vi "Get Filter Configuration String.vi"(11 "Base Filter in":refnum<class "Base Filter.lvclass">) -> (2 "Filter Configuration":string)   [LabVIEW 2016, in "Assert API Components.lvlib" / "Base Filter.lvclass"]
uses:
  Base Filter.lvclass
  Base Filter.lvclass/Base Filter.ctl
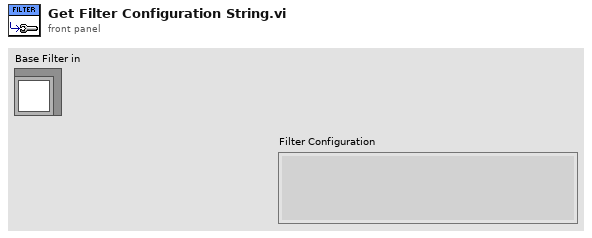
[diagram p1: front panel]
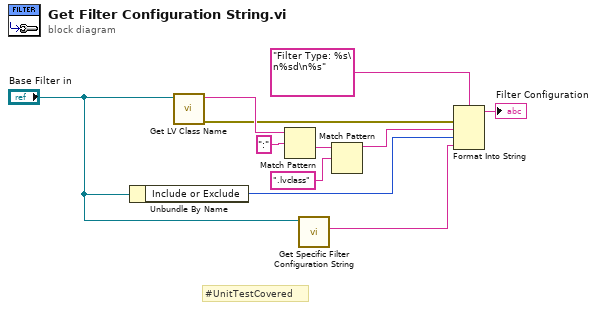
[diagram p0: block diagram]
diagram:
  # "#UnitTestCovered"
  n1 = Unbundle By Name("Base Filter in") -> ("Include or Exclude"=w3:enum16{"Include", "Exclude"})
  n2 = call <vilib>:"Get LV Class Name.vi"("object"="Base Filter in") -> ("error out"=w4:errorcluster, "class name"=w10:string)  [unwired: 9 in]
  n3 = Match Pattern(string=w10, regular expression=":") -> (after substring=w8:string)  [unwired: 1 in, 3 out]
  n4 = call-dynamic "Get Specific Filter Configuration String.vi"("Base Filter in"="Base Filter in") -> ("Filter String"=w1:string)  [unwired: 10 in]
  n5 = Match Pattern(string=w8, regular expression=".lvclass") -> (before substring=w6:string)  [unwired: 1 in, 3 out]
  n6 = Format Into String(format string="Filter Type: %s\n%sd\n%s", error in=w4, w6, w3, w1) -> (resulting string=→"Filter Configuration":string)  [unwired: 1 in, 1 out]
